vi "Server.vi"() -> ()   [LabVIEW 2020]
panel:
  out "Kitchen Door 2":bool
  out "Kitchen Door 1":bool
  out "Balcony Door 1":bool
  out "Bedroom 1 Door 1":bool
  out "Balcony Door 2":bool
  out "Bedroom 2 Door 1":bool
  out "Bedroom 1 Curtain 1":bool
  out "Bedroom 2 Curtain 1":bool
  out "Kitchen Light 1":bool
  out "Balcony Light 3":bool
  out "Balcony Light 2":bool
  out "Balcony Light 1":bool
  out "Bedroom 2 Light 1":bool
  out "Bedroom 1 Light 1":bool
  out "Master Bedroom Curtain 1":bool
  out "Master Bedroom AC 1":bool
  out "Master Bedroom Door 1":bool
  out "Master Bedroom Light 2":bool
  out "Master Bedroom Light 1":bool
  in  "Tab Control 2":enum32{"Page 1"}(tab)
  in  "WindowsMediaPlayer":refnum<k7>(container)
  out "Living Room Curtain 1":bool
  out "Living Room Door 1":bool
  in  "Tab Control":T1(tab)
  out "Light Rotation":bool
  out "Automatic Curtains":bool
  out "Time (Hour)":dbl
  out "Master Curtains":bool
  out "Master Doors":bool
  out "Master Lights":bool
  out "Adaptive Brightness":bool
  out "TV Brightness":dbl(slide) scale=0.0..6.0
  out "TV Fast Forward Reverse":bool
  out "TV Fast Forward":bool
  out "TV Channel 2":bool
  out "TV Channel 1":bool
  out "TV Pause":bool
  out "TV Play":bool
  out "TV On/Off":bool
  out "TV Volume":i32
  out "Balcony Alarm":bool
  out "Bedroom 2 Alarm":bool
  out "Bedroom 1 Alarm":bool
  out "Kitchen Alarm":bool
  out "Master Bedroom Alarm":bool
  out "Living Room Alarm":bool
  out "Living Room Temperature":dbl(slide) scale=10.0..40.0
  out "Room Brightness":dbl(slide) scale=0.0..6.0
  out "Living Room Light 1 Dim":bool
  out "Living Room Light 2 Dim":bool
  out "Master Bedroom Light 1 Dim":bool
  out "Master Bedroom Light 2 Dim":bool
  out "Master Bedroom Temperature":dbl(slide) scale=10.0..40.0
  out "Bedroom 1 Temperature":dbl(slide) scale=10.0..40.0
  out "Bedroom 1 Light 1 Dim":bool
  out "Bedroom 2 Temperature":dbl(slide) scale=10.0..40.0
  out "Bedroom 2 Light 1 Dim":bool
  out "Balcony Temperature":dbl(slide) scale=10.0..40.0
  out "Balcony Light 3 Dim":bool
  out "Balcony Light 2 Dim":bool
  out "Balcony Light 1 Dim":bool
  out "Kitchen Temperature":dbl(slide) scale=10.0..40.0
  out "Kitchen Light 1 Dim":bool
  out "Boolean":bool
  out "Living Room Light 2":bool
  out "Living Room Light 1":bool
  in  "stop":bool
  # "Server"
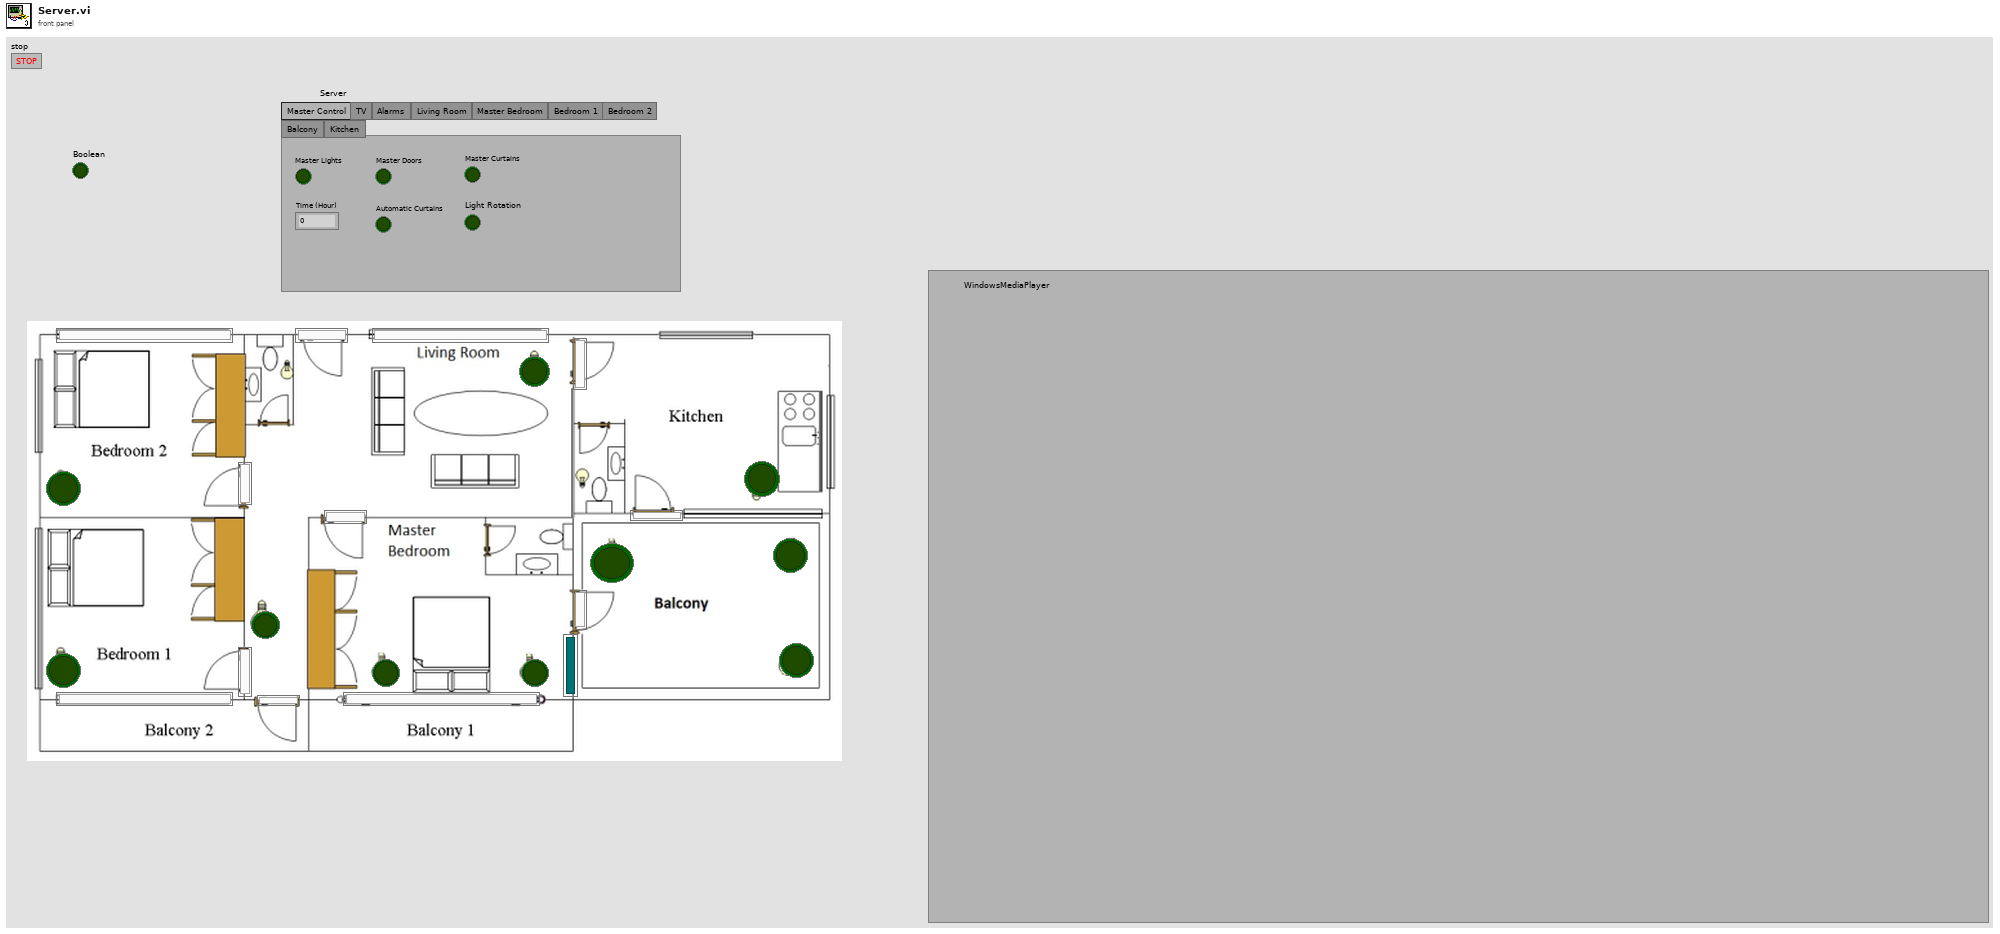
[diagram p1: front panel]
types:
  T1 = enum32{"Master Control", "TV", "Alarms", "Living Room", "Master Bedroom", "Bedroom 1", "Bedroom 2", "Balcony", "Kitchen"}
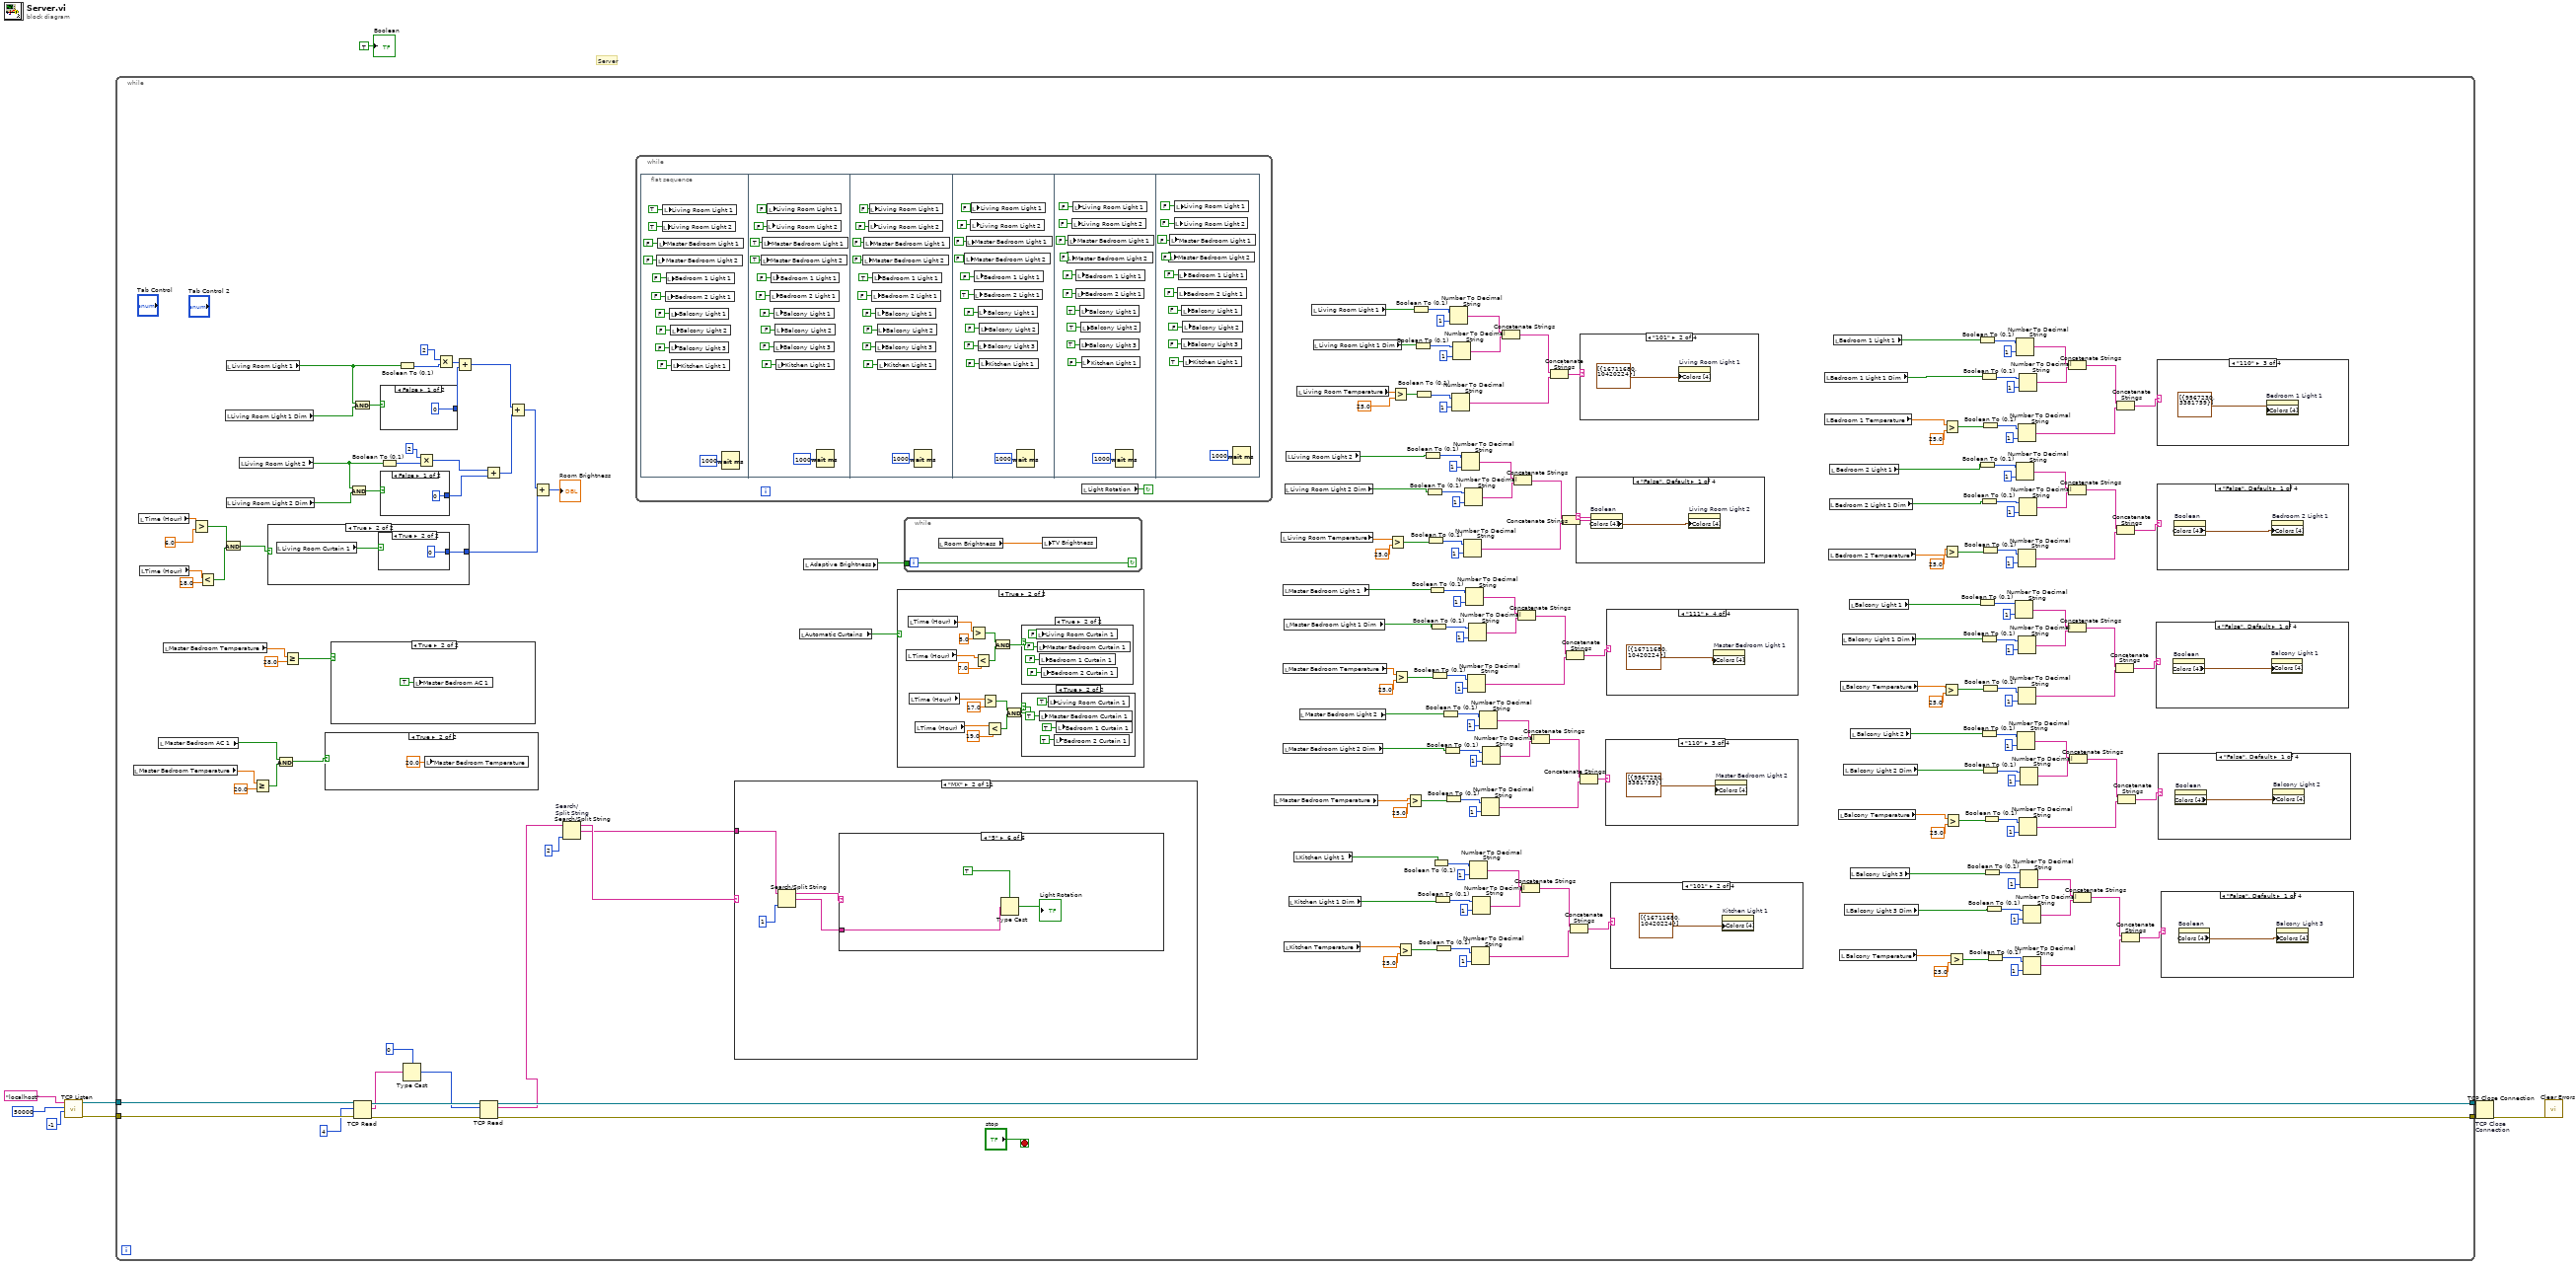
[diagram p0: block diagram]
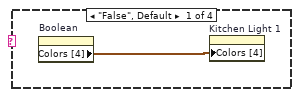
[diagram p2: hidden frame]
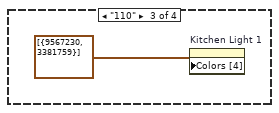
[diagram p3: hidden frame]
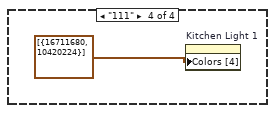
[diagram p4: hidden frame]
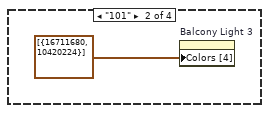
[diagram p5: hidden frame]
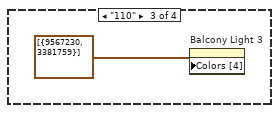
[diagram p6: hidden frame]
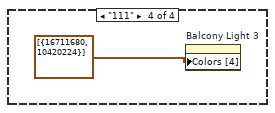
[diagram p7: hidden frame]
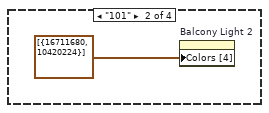
[diagram p8: hidden frame]
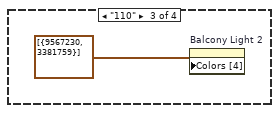
[diagram p9: hidden frame]
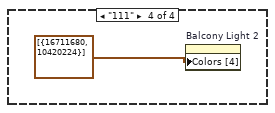
[diagram p10: hidden frame]
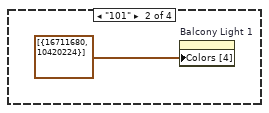
[diagram p11: hidden frame]
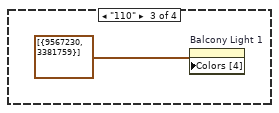
[diagram p12: hidden frame]
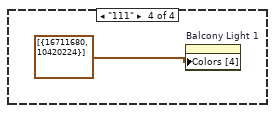
[diagram p13: hidden frame]
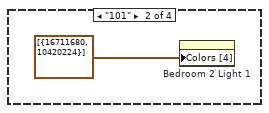
[diagram p14: hidden frame]
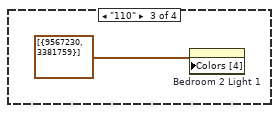
[diagram p15: hidden frame]
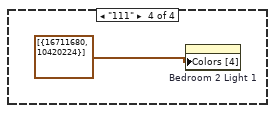
[diagram p16: hidden frame]
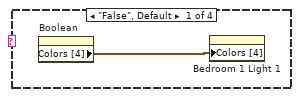
[diagram p17: hidden frame]
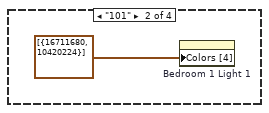
[diagram p18: hidden frame]
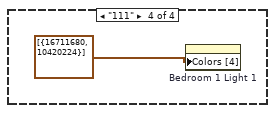
[diagram p19: hidden frame]
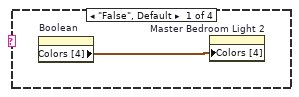
[diagram p20: hidden frame]
diagram:
  # "Server"
  n1 = call <vilib>:"TCP Listen.vi"("timeout ms (wait forever: -1)"=-1, "port"=u16 50000, "service name"="localhost") -> ("error out"=w4:errorcluster, "connection ID"=w6:refnum<k5>)  [unwired: 4 in, 3 out]
  n2 = while {
    tunnel: w6 -> [w219]
    tunnel: [w217] -> w5
    tunnel: w4 -> [w216]
    tunnel: [w214] -> w3
    stop <- "stop" stop-if-true
    n3 = local read "Master Bedroom Temperature"() -> (w141:dbl)
    n4 = local read "Time (Hour)"() -> (w154:dbl)
    n5 = local read "Time (Hour)"() -> (w152:dbl)
    n6 = local read "Master Bedroom AC 1"() -> (w142:bool)
    n7 = local read "Master Bedroom Temperature"() -> (w145:dbl)
    n8 = Greater?(x=w154, y=6.0) -> (0:w150:bool)
    n9 = Less?(x=w152, y=18.0) -> (x < y?=w149:bool)
    n10 = And(x=w150, y=w149) -> (x .and. y?=w148:bool)
    n11 = local read "Living Room Light 1 Dim"() -> (w192:bool)
    n12 = local read "Living Room Light 1"() -> (w193:bool)
    n13 = local read "Living Room Light 2 Dim"() -> (w189:bool)
    n14 = local read "Living Room Light 2"() -> (w188:bool)
    n15 = Greater Or Equal?(x=w141, y=20.0) -> (x >= y?=w139:bool)
    n16 = case shown="True" w148 {
      tunnel: [0 w347] -> w155
      frame False {
      }
      frame True {
        n17 = local read "Living Room Curtain 1"() -> (w348:bool)
        n18 = case shown="True" w348 {
          tunnel: [2 0] -> w347
          frame False {
          }
          frame True {
          }
        }
      }
    }
    n19 = And(x=w142, y=w139) -> (x .and. y?=w138:bool)
    n20 = Greater Or Equal?(x=w145, y=28.0) -> (x >= y?=w143:bool)
    n21 = case shown="True" w138 {
      frame False {
      }
      frame True {
        n22 = local write "Master Bedroom Temperature"(20.0 ("Master Bedroom Temperature")) -> ()
      }
    }
    n23 = case shown="True" w143 {
      frame False {
      }
      frame True {
        n24 = local write "Master Bedroom AC 1"(TRUE ("Master Bedroom AC 1")) -> ()
      }
    }
    n25 = And(x=w188, y=w189) -> (x .and. y?=w191:bool)
    n26 = And(x=w193, y=w192) -> (x .and. y?=w190:bool)
    n27 = TCP Read(connection ID=w219, bytes to read=4, error in (no error)=w216) -> (connection ID out=w218:refnum<k5>, data out=w212:string, error out=w215:errorcluster)  [unwired: 2 in]
    n28 = case shown="False" w190 {
      tunnel: [0 -1] -> w186
      frame False {
      }
      frame True {
      }
    }
    n29 = Boolean To (0,1)(Boolean=w188) -> (0, 1=w196:i16)
    n30 = case shown="False" w191 {
      tunnel: [0 -1] -> w187
      frame False {
      }
      frame True {
      }
    }
    n31 = Boolean To (0,1)(Boolean=w193) -> (0, 1=w198:i16)
    n32 = Type Cast(type=0 ("bytes to read"), x=w212) -> (*(type *) &x=w208:i32)
    n33 = Multiply(x=i16 2, y=w196) -> (x*y=w194:i16)
    n34 = Multiply(x=i16 2, y=w198) -> (x*y=w199:i16)
    n35 = Add(x=w199, y=w186) -> (x+y=w201:i32)
    n36 = TCP Read(connection ID=w218, bytes to read=w208, error in (no error)=w215) -> (connection ID out=w217:refnum<k5>, data out=w210:string, error out=w214:errorcluster)  [unwired: 2 in]
    n37 = Add(x=w194, y=w187) -> (x+y=w200:i32)
    n38 = Add(x=w201, y=w200) -> (x+y=w156:i32)
    n39 = Add(x=w156, y=w155) -> (x+y=→"Room Brightness":i32)
    n40 = Search/Split String "Search/\nSplit String"(string=w210, offset (0)=2) -> (substring before match=w207:string, match + rest of string=w206:string)  [unwired: 1 in, 1 out]
    n41 = while {
      stop <- w221 continue-if-true
      n42 = flat-sequence {
        frame #0 {
          n43 = local write "Master Bedroom Light 2"(FALSE ("Master Bedroom Light 2")) -> ()
          n44 = local write "Master Bedroom Light 1"(FALSE ("Master Bedroom Light 1")) -> ()
          n45 = local write "Living Room Light 2"(TRUE ("Living Room Light 2")) -> ()
          n46 = local write "Living Room Light 1"(TRUE ("Living Room Light 1")) -> ()
          n47 = local write "Bedroom 2 Light 1"(FALSE ("Bedroom 2 Light 1")) -> ()
          n48 = local write "Bedroom 1 Light 1"(FALSE ("Bedroom 1 Light 1")) -> ()
          n49 = local write "Balcony Light 1"(FALSE ("Balcony Light 1")) -> ()
          n50 = local write "Balcony Light 3"(FALSE ("Balcony Light 3")) -> ()
          n51 = local write "Balcony Light 2"(FALSE ("Balcony Light 2")) -> ()
          n52 = local write "Kitchen Light 1"(FALSE ("Kitchen Light 1")) -> ()
          n53 = Wait (ms)(milliseconds to wait=u32 1000) -> ()  [unwired: 1 out]
        }
        frame #1 {
          n54 = local write "Master Bedroom Light 2"(TRUE ("Master Bedroom Light 2")) -> ()
          n55 = local write "Master Bedroom Light 1"(TRUE ("Master Bedroom Light 1")) -> ()
          n56 = local write "Living Room Light 2"(FALSE ("Living Room Light 2")) -> ()
          n57 = local write "Living Room Light 1"(FALSE ("Living Room Light 1")) -> ()
          n58 = local write "Bedroom 2 Light 1"(FALSE ("Bedroom 2 Light 1")) -> ()
          n59 = local write "Bedroom 1 Light 1"(FALSE ("Bedroom 1 Light 1")) -> ()
          n60 = local write "Balcony Light 1"(FALSE ("Balcony Light 1")) -> ()
          n61 = local write "Balcony Light 3"(FALSE ("Balcony Light 3")) -> ()
          n62 = local write "Balcony Light 2"(FALSE ("Balcony Light 2")) -> ()
          n63 = local write "Kitchen Light 1"(FALSE ("Kitchen Light 1")) -> ()
          n64 = Wait (ms)(milliseconds to wait=u32 1000) -> ()  [unwired: 1 out]
        }
        frame #2 {
          n65 = local write "Master Bedroom Light 2"(FALSE ("Master Bedroom Light 2")) -> ()
          n66 = local write "Master Bedroom Light 1"(FALSE ("Master Bedroom Light 1")) -> ()
          n67 = local write "Living Room Light 2"(FALSE ("Living Room Light 2")) -> ()
          n68 = local write "Living Room Light 1"(FALSE ("Living Room Light 1")) -> ()
          n69 = local write "Bedroom 2 Light 1"(FALSE ("Bedroom 2 Light 1")) -> ()
          n70 = local write "Bedroom 1 Light 1"(TRUE ("Bedroom 1 Light 1")) -> ()
          n71 = local write "Balcony Light 1"(FALSE ("Balcony Light 1")) -> ()
          n72 = local write "Balcony Light 3"(FALSE ("Balcony Light 3")) -> ()
          n73 = local write "Balcony Light 2"(FALSE ("Balcony Light 2")) -> ()
          n74 = local write "Kitchen Light 1"(FALSE ("Kitchen Light 1")) -> ()
          n75 = Wait (ms)(milliseconds to wait=u32 1000) -> ()  [unwired: 1 out]
        }
        frame #3 {
          n76 = local write "Master Bedroom Light 2"(FALSE ("Master Bedroom Light 2")) -> ()
          n77 = local write "Master Bedroom Light 1"(FALSE ("Master Bedroom Light 1")) -> ()
          n78 = local write "Living Room Light 2"(FALSE ("Living Room Light 2")) -> ()
          n79 = local write "Living Room Light 1"(FALSE ("Living Room Light 1")) -> ()
          n80 = local write "Bedroom 2 Light 1"(TRUE ("Bedroom 2 Light 1")) -> ()
          n81 = local write "Bedroom 1 Light 1"(FALSE ("Bedroom 1 Light 1")) -> ()
          n82 = local write "Balcony Light 1"(FALSE ("Balcony Light 1")) -> ()
          n83 = local write "Balcony Light 3"(FALSE ("Balcony Light 3")) -> ()
          n84 = local write "Balcony Light 2"(FALSE ("Balcony Light 2")) -> ()
          n85 = local write "Kitchen Light 1"(FALSE ("Kitchen Light 1")) -> ()
          n86 = Wait (ms)(milliseconds to wait=u32 1000) -> ()  [unwired: 1 out]
        }
        frame #4 {
          n87 = local write "Master Bedroom Light 2"(FALSE ("Master Bedroom Light 2")) -> ()
          n88 = local write "Master Bedroom Light 1"(FALSE ("Master Bedroom Light 1")) -> ()
          n89 = local write "Living Room Light 2"(FALSE ("Living Room Light 2")) -> ()
          n90 = local write "Living Room Light 1"(FALSE ("Living Room Light 1")) -> ()
          n91 = local write "Bedroom 2 Light 1"(FALSE ("Bedroom 2 Light 1")) -> ()
          n92 = local write "Bedroom 1 Light 1"(FALSE ("Bedroom 1 Light 1")) -> ()
          n93 = local write "Balcony Light 1"(TRUE ("Balcony Light 1")) -> ()
          n94 = local write "Balcony Light 3"(TRUE ("Balcony Light 3")) -> ()
          n95 = local write "Balcony Light 2"(TRUE ("Balcony Light 2")) -> ()
          n96 = local write "Kitchen Light 1"(FALSE ("Kitchen Light 1")) -> ()
          n97 = Wait (ms)(milliseconds to wait=u32 1000) -> ()  [unwired: 1 out]
        }
        frame #5 {
          n98 = local write "Master Bedroom Light 2"(FALSE ("Master Bedroom Light 2")) -> ()
          n99 = local write "Master Bedroom Light 1"(FALSE ("Master Bedroom Light 1")) -> ()
          n100 = local write "Living Room Light 2"(FALSE ("Living Room Light 2")) -> ()
          n101 = local write "Living Room Light 1"(FALSE ("Living Room Light 1")) -> ()
          n102 = local write "Bedroom 2 Light 1"(FALSE ("Bedroom 2 Light 1")) -> ()
          n103 = local write "Bedroom 1 Light 1"(FALSE ("Bedroom 1 Light 1")) -> ()
          n104 = local write "Balcony Light 1"(FALSE ("Balcony Light 1")) -> ()
          n105 = local write "Balcony Light 3"(FALSE ("Balcony Light 3")) -> ()
          n106 = local write "Balcony Light 2"(FALSE ("Balcony Light 2")) -> ()
          n107 = local write "Kitchen Light 1"(TRUE ("Kitchen Light 1")) -> ()
          n108 = Wait (ms)(milliseconds to wait=u32 1000) -> ()  [unwired: 1 out]
        }
      }
      n109 = local read "Light Rotation"() -> (w221:bool)
    }
    n110 = case shown="\"MX\"" w207 {
      tunnel: w206 -> [_ w363 w387 w450 w487 w528 w556 w584 w632 w658 w685]
      frame "False", Default {
      }
      frame "MX" {
        n111 = Search/Split String(string=w363, offset (0)=1) -> (substring before match=w366:string, match + rest of string=w365:string)  [unwired: 1 in, 1 out]
        n112 = case shown="\"5\"" w366 {
          tunnel: w365 -> [_ w369 w371 w373 w377 w379]
          frame "False", Default {
          }
          frame "1" {
            n113 = Type Cast(type=TRUE, x=w369) -> (*(type *) &x=→"Master Lights":bool)
          }
          frame "2" {
            n114 = Type Cast(type=TRUE, x=w371) -> (*(type *) &x=→"Master Doors":bool)
          }
          frame "3" {
            n115 = Type Cast(type=TRUE, x=w373) -> (*(type *) &x=→"Master Curtains":bool)
          }
          frame "4" {
            n116 = Type Cast(type=TRUE, x=w377) -> (*(type *) &x=→"Automatic Curtains":bool)
          }
          frame "5" {
            n117 = Type Cast(type=TRUE, x=w379) -> (*(type *) &x=→"Light Rotation":bool)
          }
        }
      }
      frame "TV" {
        n118 = property on="WindowsMediaPlayer" class="AXCont"("Height"=u32 360 ("Container Bounds:Height")) -> ()  [unwired: 2 in, 2 out]
        n119 = property on="WindowsMediaPlayer" class="AXCont"("Width"=u32 640 ("Container Bounds:Width")) -> ()  [unwired: 2 in, 2 out]
        n120 = Search/Split String(string=w387, offset (0)=1) -> (substring before match=w386:string, match + rest of string=w385:string)  [unwired: 1 in, 1 out]
        n121 = case shown="\"1\"" w386 {
          tunnel: w385 -> [_ w390 w397 w403 w410 w418 w424 w431 w440 w442 w445]
          tunnel: "WindowsMediaPlayer" -> [_ _ w394 w402 w409 w413 w422 w430 w436 _ _]
          frame "False", Default {
          }
          frame "1" {
            n122 = Type Cast(type=TRUE, x=w390) -> (*(type *) &x=w389:bool)
            "TV On/Off" <- w389
            n123 = property on="WindowsMediaPlayer" class="AXCont"("Visible"=w389) -> ()  [unwired: 2 in, 2 out]
          }
          frame "2" {
            n124 = Automation Open(Automation Refnum=w394) -> (Automation Refnum=w395:refnum<k7>)  [unwired: 3 in, 1 out]
            n125 = property class="IWMPPlayer4"(reference=w395) -> ("controls"=w393:refnum<k7>)  [unwired: 1 in, 2 out]
            n126 = Type Cast(type=TRUE, x=w397) -> (*(type *) &x=→"TV Play":bool)
            n127 = invoke class="IWMPControls" method="play"(reference=w393) -> (reference out=w392:refnum<k7>)  [unwired: 2 in, 2 out]
            n128 = Close Reference(reference=w392) -> ()  [unwired: 1 in, 1 out]
          }
          frame "3" {
            n129 = Automation Open(Automation Refnum=w402) -> (Automation Refnum=w401:refnum<k7>)  [unwired: 3 in, 1 out]
            n130 = property class="IWMPPlayer4"(reference=w401) -> ("controls"=w400:refnum<k7>)  [unwired: 1 in, 2 out]
            n131 = Type Cast(type=TRUE, x=w403) -> (*(type *) &x=→"TV Pause":bool)
            n132 = invoke class="IWMPControls" method="pause"(reference=w400) -> (reference out=w399:refnum<k7>)  [unwired: 2 in, 2 out]
            n133 = Close Reference(reference=w399) -> ()  [unwired: 1 in, 1 out]
          }
          frame "4" {
            n134 = Automation Open(Automation Refnum=w409) -> (Automation Refnum=w408:refnum<k7>)  [unwired: 3 in, 1 out]
            n135 = property class="IWMPPlayer4"(reference=w408, "URL"="C:/Ah ! Guilty Gear !!.mp4") -> (reference out=w407:refnum<k7>)  [unwired: 1 in, 1 out]
            n136 = Type Cast(type=TRUE, x=w410) -> (*(type *) &x=→"TV Channel 1":bool)
            n137 = Close Reference(reference=w407) -> ()  [unwired: 1 in, 1 out]
          }
          frame "5" {
            n138 = Automation Open(Automation Refnum=w413) -> (Automation Refnum=w414:refnum<k7>)  [unwired: 3 in, 1 out]
            n139 = property class="IWMPPlayer4"(reference=w414, "URL"="C:/TIME2REALIZE.mp4") -> (reference out=w415:refnum<k7>)  [unwired: 1 in, 1 out]
            n140 = Type Cast(type=TRUE, x=w418) -> (*(type *) &x=→"TV Channel 2":bool)
            n141 = Close Reference(reference=w415) -> ()  [unwired: 1 in, 1 out]
          }
          frame "6" {
            n142 = Automation Open(Automation Refnum=w422) -> (Automation Refnum=w421:refnum<k7>)  [unwired: 3 in, 1 out]
            n143 = property class="IWMPPlayer4"(reference=w421) -> ("controls"=w423:refnum<k7>)  [unwired: 1 in, 2 out]
            n144 = Type Cast(type=TRUE, x=w424) -> (*(type *) &x=→"TV Fast Forward":bool)
            n145 = invoke class="IWMPControls" method="fastForward"(reference=w423) -> (reference out=w420:refnum<k7>)  [unwired: 2 in, 2 out]
            n146 = Close Reference(reference=w420) -> ()  [unwired: 1 in, 1 out]
          }
          frame "7" {
            n147 = Automation Open(Automation Refnum=w430) -> (Automation Refnum=w429:refnum<k7>)  [unwired: 3 in, 1 out]
            n148 = property class="IWMPPlayer4"(reference=w429) -> ("controls"=w428:refnum<k7>)  [unwired: 1 in, 2 out]
            n149 = Type Cast(type=TRUE, x=w431) -> (*(type *) &x=→"TV Fast Forward Reverse":bool)
            n150 = invoke class="IWMPControls" method="fastReverse"(reference=w428) -> (reference out=w427:refnum<k7>)  [unwired: 2 in, 2 out]
            n151 = Close Reference(reference=w427) -> ()  [unwired: 1 in, 1 out]
          }
          frame "8" {
            n152 = Automation Open(Automation Refnum=w436) -> (Automation Refnum=w435:refnum<k7>)  [unwired: 3 in, 1 out]
            n153 = property class="IWMPPlayer4"(reference=w435) -> ("settings"=w437:refnum<k7>)  [unwired: 1 in, 2 out]
            n154 = Type Cast(type=0, x=w440) -> (*(type *) &x=w438:i32)
            "TV Volume" <- w438
            n155 = property class="IWMPSettings"(reference=w437, "volume"=w438) -> (reference out=w434:refnum<k7>)  [unwired: 1 in, 1 out]
            n156 = Close Reference(reference=w434) -> ()  [unwired: 1 in, 1 out]
          }
          frame "9" {
            n157 = Type Cast(type=0.0, x=w442) -> (*(type *) &x=→"TV Brightness":dbl)
          }
          frame "10" {
            n158 = Type Cast(type=TRUE, x=w445) -> (*(type *) &x=→"Adaptive Brightness":bool)
          }
        }
      }
      frame "LR" {
        n159 = Search/Split String(string=w450, offset (0)=1) -> (substring before match=w448:string, match + rest of string=w447:string)  [unwired: 1 in, 1 out]
        n160 = case shown="\"1\"" w448 {
          tunnel: w447 -> [_ w453 w460 w466 w469 w473 w480]
          frame "False", Default {
          }
          frame "1" {
            n161 = local read "Master Lights"() -> (w452:bool)
            n162 = Not(x=w452) -> (.not. x?=w451:bool)
            n163 = case shown="True" w451 {
              tunnel: w453 -> [_ w455]
              frame False {
                n164 = local write "Living Room Alarm"(TRUE ("Living Room Alarm")) -> ()
              }
              frame True {
                n165 = Type Cast(type=FALSE ("Boolean"), x=w455) -> (*(type *) &x=→"Living Room Light 1":bool)
              }
            }
          }
          frame "2" {
            n166 = local read "Master Lights"() -> (w459:bool)
            n167 = Not(x=w459) -> (.not. x?=w458:bool)
            n168 = case shown="True" w458 {
              tunnel: w460 -> [_ w462]
              frame False {
                n169 = local write "Living Room Alarm"(TRUE ("Living Room Alarm")) -> ()
              }
              frame True {
                n170 = Type Cast(type=FALSE ("Boolean"), x=w462) -> (*(type *) &x=→"Living Room Light 2":bool)
              }
            }
          }
          frame "3" {
            n171 = Type Cast(type=FALSE ("Boolean"), x=w466) -> (*(type *) &x=→"Living Room Light 1 Dim":bool)
          }
          frame "4" {
            n172 = Type Cast(type=FALSE ("Boolean"), x=w469) -> (*(type *) &x=→"Living Room Light 2 Dim":bool)
          }
          frame "5" {
            n173 = local read "Master Curtains"() -> (w472:bool)
            n174 = Not(x=w472) -> (.not. x?=w471:bool)
            n175 = case shown="True" w471 {
              tunnel: w473 -> [_ w477]
              frame False {
                n176 = local write "Living Room Alarm"(TRUE ("Living Room Alarm")) -> ()
              }
              frame True {
                n177 = Type Cast(type=TRUE, x=w477) -> (*(type *) &x=→"Living Room Curtain 1":bool)
              }
            }
          }
          frame "6" {
            n178 = local read "Master Doors"() -> (w479:bool)
            n179 = Not(x=w479) -> (.not. x?=w478:bool)
            n180 = case shown="False" w478 {
              tunnel: w480 -> [_ w482]
              frame False {
                n181 = local write "Living Room Alarm"(TRUE ("Living Room Alarm")) -> ()
              }
              frame True {
                n182 = Type Cast(type=FALSE ("Boolean"), x=w482) -> (*(type *) &x=→"Living Room Door 1":bool)
              }
            }
          }
        }
      }
      frame "MB" {
        n183 = Search/Split String(string=w487, offset (0)=1) -> (substring before match=w486:string, match + rest of string=w485:string)  [unwired: 1 in, 1 out]
        n184 = case shown="\"5\"" w486 {
          tunnel: w485 -> [_ w489 w498 w504 w507 w511 w516 w524]
          frame "False", Default {
          }
          frame "1" {
            n185 = local read "Master Lights"() -> (w491:bool)
            n186 = Not(x=w491) -> (.not. x?=w490:bool)
            n187 = case shown="True" w490 {
              tunnel: w489 -> [_ w494]
              frame False {
                n188 = local write "Master Bedroom Alarm"(TRUE ("Master Bedroom Alarm")) -> ()
              }
              frame True {
                n189 = Type Cast(type=FALSE ("Boolean"), x=w494) -> (*(type *) &x=→"Master Bedroom Light 1":bool)
              }
            }
          }
          frame "2" {
            n190 = local read "Master Lights"() -> (w497:bool)
            n191 = Not(x=w497) -> (.not. x?=w496:bool)
            n192 = case shown="False" w496 {
              tunnel: w498 -> [_ w501]
              frame False {
                n193 = local write "Master Bedroom Alarm"(TRUE ("Master Bedroom Alarm")) -> ()
              }
              frame True {
                n194 = Type Cast(type=FALSE ("Boolean"), x=w501) -> (*(type *) &x=→"Master Bedroom Light 2":bool)
              }
            }
          }
          frame "3" {
            n195 = Type Cast(type=FALSE ("Boolean"), x=w504) -> (*(type *) &x=→"Master Bedroom Light 1 Dim":bool)
          }
          frame "4" {
            n196 = Type Cast(type=FALSE ("Boolean"), x=w507) -> (*(type *) &x=→"Master Bedroom Light 2 Dim":bool)
          }
          frame "5" {
            n197 = local read "Master Curtains"() -> (w510:bool)
            n198 = Not(x=w510) -> (.not. x?=w509:bool)
            n199 = case shown="True" w509 {
              tunnel: w511 -> [_ w514]
              frame False {
                n200 = local write "Master Bedroom Alarm"(TRUE ("Master Bedroom Alarm")) -> ()
              }
              frame True {
                n201 = Type Cast(type=FALSE ("Boolean"), x=w514) -> (*(type *) &x=→"Master Bedroom Curtain 1":bool)
              }
            }
          }
          frame "6" {
            n202 = local read "Master Doors"() -> (w518:bool)
            n203 = Not(x=w518) -> (.not. x?=w517:bool)
            n204 = case shown="True" w517 {
              tunnel: w516 -> [_ w521]
              frame False {
                n205 = local write "Master Bedroom Alarm"(TRUE ("Master Bedroom Alarm")) -> ()
              }
              frame True {
                n206 = Type Cast(type=FALSE ("Boolean"), x=w521) -> (*(type *) &x=→"Master Bedroom Door 1":bool)
              }
            }
          }
          frame "7" {
            n207 = Type Cast(type=FALSE ("Boolean"), x=w524) -> (*(type *) &x=→"Master Bedroom AC 1":bool)
          }
        }
      }
      frame "B1" {
        n208 = Search/Split String(string=w528, offset (0)=1) -> (substring before match=w527:string, match + rest of string=w526:string)  [unwired: 1 in, 1 out]
        n209 = case shown="\"3\"" w527 {
          tunnel: w526 -> [_ w532 w538 w540 w547]
          frame "False", Default {
          }
          frame "1" {
            n210 = local read "Master Lights"() -> (w531:bool)
            n211 = Not(x=w531) -> (.not. x?=w530:bool)
            n212 = case shown="True" w530 {
              tunnel: w532 -> [_ w534]
              frame False {
                n213 = local write "Bedroom 1 Alarm"(TRUE ("Bedroom 1 Alarm")) -> ()
              }
              frame True {
                n214 = Type Cast(type=TRUE, x=w534) -> (*(type *) &x=→"Bedroom 1 Light 1":bool)
              }
            }
          }
          frame "2" {
            n215 = Type Cast(type=TRUE, x=w538) -> (*(type *) &x=→"Bedroom 1 Light 1 Dim":bool)
          }
          frame "3" {
            n216 = local read "Master Curtains"() -> (w542:bool)
            n217 = Not(x=w542) -> (.not. x?=w541:bool)
            n218 = case shown="True" w541 {
              tunnel: w540 -> [_ w544]
              frame False {
                n219 = local write "Bedroom 1 Alarm"(TRUE ("Bedroom 1 Alarm")) -> ()
              }
              frame True {
                n220 = Type Cast(type=FALSE ("Boolean"), x=w544) -> (*(type *) &x=→"Bedroom 1 Curtain 1":bool)
              }
            }
          }
          frame "4" {
            n221 = local read "Master Doors"() -> (w548:bool)
            n222 = Not(x=w548) -> (.not. x?=w549:bool)
            n223 = case shown="False" w549 {
              tunnel: w547 -> [_ w551]
              frame False {
                n224 = local write "Bedroom 1 Alarm"(TRUE ("Bedroom 1 Alarm")) -> ()
              }
              frame True {
                n225 = Type Cast(type=FALSE ("Boolean"), x=w551) -> (*(type *) &x=→"Bedroom 1 Door 1":bool)
              }
            }
          }
        }
      }
      frame "B2" {
        n226 = Search/Split String(string=w556, offset (0)=1) -> (substring before match=w555:string, match + rest of string=w554:string)  [unwired: 1 in, 1 out]
        n227 = case shown="\"4\"" w555 {
          tunnel: w554 -> [_ w560 w565 w568 w577]
          frame "False", Default {
          }
          frame "1" {
            n228 = local read "Master Lights"() -> (w558:bool)
            n229 = Not(x=w558) -> (.not. x?=w559:bool)
            n230 = case shown="True" w559 {
              tunnel: w560 -> [_ w563]
              frame False {
                n231 = local write "Bedroom 2 Alarm"(TRUE ("Bedroom 2 Alarm")) -> ()
              }
              frame True {
                n232 = Type Cast(type=TRUE, x=w563) -> (*(type *) &x=→"Bedroom 2 Light 1":bool)
              }
            }
          }
          frame "2" {
            n233 = Type Cast(type=TRUE, x=w565) -> (*(type *) &x=→"Bedroom 2 Light 1 Dim":bool)
          }
          frame "3" {
            n234 = local read "Master Curtains"() -> (w570:bool)
            n235 = Not(x=w570) -> (.not. x?=w569:bool)
            n236 = case shown="False" w569 {
              tunnel: w568 -> [_ w572]
              frame False {
                n237 = local write "Bedroom 2 Alarm"(TRUE ("Bedroom 2 Alarm")) -> ()
              }
              frame True {
                n238 = Type Cast(type=FALSE ("Boolean"), x=w572) -> (*(type *) &x=→"Bedroom 2 Curtain 1":bool)
              }
            }
          }
          frame "4" {
            n239 = local read "Master Doors"() -> (w576:bool)
            n240 = Not(x=w576) -> (.not. x?=w575:bool)
            n241 = case shown="False" w575 {
              tunnel: w577 -> [_ w579]
              frame False {
                n242 = local write "Bedroom 2 Alarm"(TRUE ("Bedroom 2 Alarm")) -> ()
              }
              frame True {
                n243 = Type Cast(type=FALSE ("Boolean"), x=w579) -> (*(type *) &x=→"Bedroom 2 Door 1":bool)
              }
            }
          }
        }
      }
      frame "BA" {
        n244 = Search/Split String(string=w584, offset (0)=1) -> (substring before match=w583:string, match + rest of string=w582:string)  [unwired: 1 in, 1 out]
        n245 = case shown="\"1\"" w583 {
          tunnel: w582 -> [_ w588 w595 w602 w607 w610 w613 w618 w625]
          frame "False", Default {
          }
          frame "1" {
            n246 = local read "Master Lights"() -> (w586:bool)
            n247 = Not(x=w586) -> (.not. x?=w587:bool)
            n248 = case shown="True" w587 {
              tunnel: w588 -> [_ w590]
              frame False {
                n249 = local write "Balcony Alarm"(TRUE ("Balcony Alarm")) -> ()
              }
              frame True {
                n250 = Type Cast(type=TRUE, x=w590) -> (*(type *) &x=→"Balcony Light 1":bool)
              }
            }
          }
          frame "2" {
            n251 = local read "Master Lights"() -> (w594:bool)
            n252 = Not(x=w594) -> (.not. x?=w593:bool)
            n253 = case shown="False" w593 {
              tunnel: w595 -> [_ w597]
              frame False {
                n254 = local write "Balcony Alarm"(TRUE ("Balcony Alarm")) -> ()
              }
              frame True {
                n255 = Type Cast(type=TRUE, x=w597) -> (*(type *) &x=→"Balcony Light 2":bool)
              }
            }
          }
          frame "3" {
            n256 = local read "Master Lights"() -> (w600:bool)
            n257 = Not(x=w600) -> (.not. x?=w601:bool)
            n258 = case shown="False" w601 {
              tunnel: w602 -> [_ w604]
              frame False {
                n259 = local write "Balcony Alarm"(TRUE ("Balcony Alarm")) -> ()
              }
              frame True {
                n260 = Type Cast(type=TRUE, x=w604) -> (*(type *) &x=→"Balcony Light 3":bool)
              }
            }
          }
          frame "4" {
            n261 = Type Cast(type=FALSE ("Boolean"), x=w607) -> (*(type *) &x=→"Balcony Light 1 Dim":bool)
          }
          frame "5" {
            n262 = Type Cast(type=FALSE ("Boolean"), x=w610) -> (*(type *) &x=→"Balcony Light 2 Dim":bool)
          }
          frame "6" {
            n263 = Type Cast(type=FALSE ("Boolean"), x=w613) -> (*(type *) &x=→"Balcony Light 3 Dim":bool)
          }
          frame "7" {
            n264 = local read "Master Doors"() -> (w617:bool)
            n265 = Not(x=w617) -> (.not. x?=w616:bool)
            n266 = case shown="False" w616 {
              tunnel: w618 -> [_ w620]
              frame False {
                n267 = local write "Balcony Alarm"(TRUE) -> ()
              }
              frame True {
                n268 = Type Cast(type=FALSE ("Boolean"), x=w620) -> (*(type *) &x=→"Balcony Door 1":bool)
              }
            }
          }
          frame "8" {
            n269 = local read "Balcony Alarm"() -> (w624:bool)
            n270 = Not(x=w624) -> (.not. x?=w623:bool)
            n271 = case shown="False" w623 {
              tunnel: w625 -> [_ w627]
              frame False {
                n272 = local write "Balcony Alarm"(TRUE ("Balcony Alarm")) -> ()
              }
              frame True {
                n273 = Type Cast(type=FALSE ("Boolean"), x=w627) -> (*(type *) &x=→"Balcony Door 2":bool)
              }
            }
          }
        }
      }
      frame "KI" {
        n274 = Search/Split String(string=w632, offset (0)=1) -> (substring before match=w631:string, match + rest of string=w630:string)  [unwired: 1 in, 1 out]
        n275 = case shown="\"1\"" w631 {
          tunnel: w630 -> [_ w636 w642 w646 w653]
          frame "False", Default {
          }
          frame "1" {
            n276 = local read "Master Lights"() -> (w635:bool)
            n277 = Not(x=w635) -> (.not. x?=w634:bool)
            n278 = case shown="True" w634 {
              tunnel: w636 -> [_ w638]
              frame False {
                n279 = local write "Kitchen Alarm"(TRUE ("Kitchen Alarm")) -> ()
              }
              frame True {
                n280 = Type Cast(type=TRUE, x=w638) -> (*(type *) &x=→"Kitchen Light 1":bool)
              }
            }
          }
          frame "2" {
            n281 = Type Cast(type=FALSE ("Boolean"), x=w642) -> (*(type *) &x=→"Kitchen Light 1 Dim":bool)
          }
          frame "3" {
            n282 = local read "Master Doors"() -> (w645:bool)
            n283 = Not(x=w645) -> (.not. x?=w644:bool)
            n284 = case shown="False" w644 {
              tunnel: w646 -> [_ w648]
              frame False {
                n285 = local write "Kitchen Alarm"(TRUE ("Kitchen Alarm")) -> ()
              }
              frame True {
                n286 = Type Cast(type=FALSE ("Boolean"), x=w648) -> (*(type *) &x=→"Kitchen Door 1":bool)
              }
            }
          }
          frame "4" {
            n287 = local read "Master Doors"() -> (w652:bool)
            n288 = Not(x=w652) -> (.not. x?=w651:bool)
            n289 = case shown="False" w651 {
              tunnel: w653 -> [_ w655]
              frame False {
                n290 = local write "Kitchen Alarm"(TRUE ("Kitchen Alarm")) -> ()
              }
              frame True {
                n291 = Type Cast(type=FALSE ("Boolean"), x=w655) -> (*(type *) &x=→"Kitchen Door 2":bool)
              }
            }
          }
        }
      }
      frame "HX" {
        n292 = Search/Split String(string=w658, offset (0)=1) -> (substring before match=w660:string, match + rest of string=w661:string)  [unwired: 1 in, 1 out]
        n293 = case shown="\"4\"" w660 {
          tunnel: w661 -> [_ w662 w666 w669 w671 w674 w677 w680]
          frame "False", Default {
          }
          frame "1" {
            n294 = Type Cast(type=0.0, x=w662) -> (*(type *) &x=→"Living Room Temperature":dbl)
          }
          frame "2" {
            n295 = Type Cast(type=0.0, x=w666) -> (*(type *) &x=→"Time (Hour)":dbl)
          }
          frame "3" {
            n296 = Type Cast(type=0.0, x=w669) -> (*(type *) &x=→"Master Bedroom Temperature":dbl)
          }
          frame "4" {
            n297 = Type Cast(type=0.0, x=w671) -> (*(type *) &x=→"Bedroom 1 Temperature":dbl)
          }
          frame "5" {
            n298 = Type Cast(type=0.0, x=w674) -> (*(type *) &x=→"Bedroom 2 Temperature":dbl)
          }
          frame "6" {
            n299 = Type Cast(type=0.0, x=w677) -> (*(type *) &x=→"Balcony Temperature":dbl)
          }
          frame "7" {
            n300 = Type Cast(type=0.0, x=w680) -> (*(type *) &x=→"Kitchen Temperature":dbl)
          }
        }
      }
      frame "AL" {
        n301 = Search/Split String(string=w685, offset (0)=1) -> (substring before match=w684:string, match + rest of string=w683:string)  [unwired: 1 in, 1 out]
        n302 = case shown="\"6\"" w684 {
          tunnel: w683 -> [_ w688 w691 w694 w696 w700 w702]
          frame "False", Default {
          }
          frame "1" {
            n303 = Type Cast(type=TRUE, x=w688) -> (*(type *) &x=→"Living Room Alarm":bool)
          }
          frame "2" {
            n304 = Type Cast(type=FALSE ("Boolean"), x=w691) -> (*(type *) &x=→"Master Bedroom Alarm":bool)
          }
          frame "3" {
            n305 = Type Cast(type=FALSE ("Boolean"), x=w694) -> (*(type *) &x=→"Bedroom 1 Alarm":bool)
          }
          frame "4" {
            n306 = Type Cast(type=FALSE ("Boolean"), x=w696) -> (*(type *) &x=→"Bedroom 2 Alarm":bool)
          }
          frame "5" {
            n307 = Type Cast(type=FALSE ("Boolean"), x=w700) -> (*(type *) &x=→"Balcony Alarm":bool)
          }
          frame "6" {
            n308 = Type Cast(type=FALSE ("Boolean"), x=w702) -> (*(type *) &x=→"Kitchen Alarm":bool)
          }
        }
      }
    }
    n309 = local read "Automatic Curtains"() -> (w147:bool)
    n310 = local read "Adaptive Brightness"() -> (w146:bool)
    n311 = case shown="True" w147 {
      frame False {
      }
      frame True {
        n312 = local read "Time (Hour)"() -> (w335:dbl)
        n313 = local read "Time (Hour)"() -> (w337:dbl)
        n314 = local read "Time (Hour)"() -> (w324:dbl)
        n315 = local read "Time (Hour)"() -> (w325:dbl)
        n316 = Greater?(x=w337, y=5.0) -> (0:w333:bool)
        n317 = Less?(x=w335, y=7.0) -> (x < y?=w332:bool)
        n318 = Greater?(x=w324, y=17.0) -> (0:w328:bool)
        n319 = Less?(x=w325, y=19.0) -> (x < y?=w327:bool)
        n320 = And(x=w333, y=w332) -> (x .and. y?=w331:bool)
        n321 = And(x=w328, y=w327) -> (x .and. y?=w326:bool)
        n322 = case shown="True" w331 {
          frame False {
          }
          frame True {
            n323 = local write "Living Room Curtain 1"(FALSE ("Living Room Curtain")) -> ()
            n324 = local write "Master Bedroom Curtain 1"(FALSE ("Master Bedroom Curtain 1")) -> ()
            n325 = local write "Bedroom 1 Curtain 1"(FALSE ("Bedroom 1 Curtain 1")) -> ()
            n326 = local write "Bedroom 2 Curtain 1"(FALSE ("Bedroom 2 Curtain 1")) -> ()
          }
        }
        n327 = case shown="True" w326 {
          frame False {
          }
          frame True {
            n328 = local write "Master Bedroom Curtain 1"(TRUE ("Master Bedroom Curtain 1")) -> ()
            n329 = local write "Living Room Curtain 1"(TRUE ("Living Room Curtain")) -> ()
            n330 = local write "Bedroom 2 Curtain 1"(TRUE ("Bedroom 2 Curtain 1")) -> ()
            n331 = local write "Bedroom 1 Curtain 1"(TRUE ("Bedroom 1 Curtain 1")) -> ()
          }
        }
      }
    }
    n332 = while {
      tunnel: w146 -> [w323]
      stop <- w323 continue-if-true
      n333 = local read "Room Brightness"() -> (w322:dbl)
      n334 = local write "TV Brightness"(w322) -> ()
    }
    n335 = local read "Master Bedroom Temperature"() -> (w93:dbl)
    n336 = local read "Living Room Temperature"() -> (w204:dbl)
    n337 = local read "Master Bedroom Light 1"() -> (w96:bool)
    n338 = local read "Master Bedroom Temperature"() -> (w98:dbl)
    n339 = local read "Master Bedroom Light 2 Dim"() -> (w94:bool)
    n340 = local read "Master Bedroom Light 1 Dim"() -> (w97:bool)
    n341 = local read "Kitchen Temperature"() -> (w24:dbl)
    n342 = local read "Living Room Light 2 Dim"() -> (w160:bool)
    n343 = local read "Living Room Light 2"() -> (w161:bool)
    n344 = local read "Kitchen Light 1 Dim"() -> (w23:bool)
    n345 = local read "Kitchen Light 1"() -> (w22:bool)
    n346 = local read "Living Room Temperature"() -> (w202:dbl)
    n347 = local read "Master Bedroom Light 2"() -> (w95:bool)
    n348 = local read "Living Room Light 1"() -> (w183:bool)
    n349 = local read "Living Room Light 1 Dim"() -> (w185:bool)
    n350 = Greater?(x=w204, y=25.0) -> (0:w159:bool)
    n351 = Greater?(x=w202, y=25.0) -> (0:w184:bool)
    n352 = Greater?(x=w98, y=25.0) -> (0:w126:bool)
    n353 = Greater?(x=w24, y=25.0) -> (0:w26:bool)
    n354 = Greater?(x=w93, y=25.0) -> (0:w114:bool)
    n355 = Boolean To (0,1)(Boolean=w183) -> (0, 1=w178:i16)
    n356 = Boolean To (0,1)(Boolean=w185) -> (0, 1=w181:i16)
    n357 = Boolean To (0,1)(Boolean=w184) -> (0, 1=w177:i16)
    n358 = Boolean To (0,1)(Boolean=w161) -> (0, 1=w167:i16)
    n359 = Boolean To (0,1)(Boolean=w160) -> (0, 1=w170:i16)
    n360 = Boolean To (0,1)(Boolean=w159) -> (0, 1=w166:i16)
    n361 = Boolean To (0,1)(Boolean=w96) -> (0, 1=w132:i16)
    n362 = Boolean To (0,1)(Boolean=w97) -> (0, 1=w135:i16)
    n363 = Boolean To (0,1)(Boolean=w126) -> (0, 1=w131:i16)
    n364 = Boolean To (0,1)(Boolean=w22) -> (0, 1=w32:i16)
    n365 = Boolean To (0,1)(Boolean=w23) -> (0, 1=w35:i16)
    n366 = Boolean To (0,1)(Boolean=w26) -> (0, 1=w31:i16)
    n367 = Boolean To (0,1)(Boolean=w95) -> (0, 1=w120:i16)
    n368 = Boolean To (0,1)(Boolean=w94) -> (0, 1=w123:i16)
    n369 = Boolean To (0,1)(Boolean=w114) -> (0, 1=w119:i16)
    n370 = Number To Decimal String(number=w178, width (-)=i16 1) -> (decimal integer string=w175:string)
    n371 = Number To Decimal String(number=w177, width (-)=i16 1) -> (decimal integer string=w173:string)
    n372 = Number To Decimal String(number=w181, width (-)=i16 1) -> (decimal integer string=w176:string)
    n373 = Number To Decimal String(number=w167, width (-)=i16 1) -> (decimal integer string=w164:string)
    n374 = Number To Decimal String(number=w166, width (-)=i16 1) -> (decimal integer string=w162:string)
    n375 = Number To Decimal String(number=w170, width (-)=i16 1) -> (decimal integer string=w165:string)
    n376 = Number To Decimal String(number=w132, width (-)=i16 1) -> (decimal integer string=w129:string)
    n377 = Number To Decimal String(number=w131, width (-)=i16 1) -> (decimal integer string=w127:string)
    n378 = Number To Decimal String(number=w135, width (-)=i16 1) -> (decimal integer string=w130:string)
    n379 = Number To Decimal String(number=w32, width (-)=i16 1) -> (decimal integer string=w29:string)
    n380 = Number To Decimal String(number=w31, width (-)=i16 1) -> (decimal integer string=w27:string)
    n381 = Number To Decimal String(number=w35, width (-)=i16 1) -> (decimal integer string=w30:string)
    n382 = Number To Decimal String(number=w120, width (-)=i16 1) -> (decimal integer string=w117:string)
    n383 = Number To Decimal String(number=w119, width (-)=i16 1) -> (decimal integer string=w115:string)
    n384 = Number To Decimal String(number=w123, width (-)=i16 1) -> (decimal integer string=w118:string)
    n385 = Concatenate Strings(w175, w176) -> (w174:string)
    n386 = Concatenate Strings(w164, w165) -> (w163:string)
    n387 = Concatenate Strings(w129, w130) -> (w128:string)
    n388 = Concatenate Strings(w29, w30) -> (w28:string)
    n389 = Concatenate Strings(w117, w118) -> (w116:string)
    n390 = Concatenate Strings(w174, w173) -> (w172:string)
    n391 = Concatenate Strings(w163, w162) -> (w158:string)
    n392 = Concatenate Strings(w128, w127) -> (w112:string)
    n393 = Concatenate Strings(w28, w27) -> (w25:string)
    n394 = case shown="\"False\", Default" w158 {
      frame "False", Default {
        n395 = property on="Boolean" class="Bool (strict)"() -> ("Colors [4]"=w351:cluster{u32, u32}[])  [unwired: 2 in, 2 out]
        n396 = property on="Living Room Light 2" class="Bool (strict)"("Colors [4]"=w351) -> ()  [unwired: 2 in, 2 out]
      }
      frame "101" {
        n397 = property on="Living Room Light 2" class="Bool (strict)"("Colors [4]"=cluster{u32, u32}[] [{16711680, 10420224}]) -> ()  [unwired: 2 in, 2 out]
      }
      frame "110" {
        n398 = property on="Living Room Light 2" class="Bool (strict)"("Colors [4]"=cluster{u32, u32}[] [{9567230, 3381759}]) -> ()  [unwired: 2 in, 2 out]
      }
      frame "111" {
        n399 = property on="Living Room Light 2" class="Bool (strict)"("Colors [4]"=cluster{u32, u32}[] [{16711680, 10420224}]) -> ()  [unwired: 2 in, 2 out]
      }
    }
    n400 = case shown="\"101\"" w172 {
      frame "False", Default {
        n401 = property on="Boolean" class="Bool (strict)"() -> ("Colors [4]"=w355:cluster{u32, u32}[])  [unwired: 2 in, 2 out]
        n402 = property on="Living Room Light 1" class="Bool (strict)"("Colors [4]"=w355) -> ()  [unwired: 2 in, 2 out]
      }
      frame "101" {
        n403 = property on="Living Room Light 1" class="Bool (strict)"("Colors [4]"=cluster{u32, u32}[] [{16711680, 10420224}]) -> ()  [unwired: 2 in, 2 out]
      }
      frame "110" {
        n404 = property on="Living Room Light 1" class="Bool (strict)"("Colors [4]"=cluster{u32, u32}[] [{9567230, 3381759}]) -> ()  [unwired: 2 in, 2 out]
      }
      frame "111" {
        n405 = property on="Living Room Light 1" class="Bool (strict)"("Colors [4]"=cluster{u32, u32}[] [{16711680, 10420224}]) -> ()  [unwired: 2 in, 2 out]
      }
    }
    n406 = Concatenate Strings(w116, w115) -> (w113:string)
    n407 = case shown="\"110\"" w113 {
      frame "False", Default {
        n408 = property on="Boolean" class="Bool (strict)"() -> ("Colors [4]"=w312:cluster{u32, u32}[])  [unwired: 2 in, 2 out]
        n409 = property on="Master Bedroom Light 2" class="Bool (strict)"("Colors [4]"=w312) -> ()  [unwired: 2 in, 2 out]
      }
      frame "101" {
        n410 = property on="Master Bedroom Light 2" class="Bool (strict)"("Colors [4]"=cluster{u32, u32}[] [{16711680, 10420224}]) -> ()  [unwired: 2 in, 2 out]
      }
      frame "110" {
        n411 = property on="Master Bedroom Light 2" class="Bool (strict)"("Colors [4]"=cluster{u32, u32}[] [{9567230, 3381759}]) -> ()  [unwired: 2 in, 2 out]
      }
      frame "111" {
        n412 = property on="Master Bedroom Light 2" class="Bool (strict)"("Colors [4]"=cluster{u32, u32}[] [{16711680, 10420224}]) -> ()  [unwired: 2 in, 2 out]
      }
    }
    n413 = case shown="\"111\"" w112 {
      frame "False", Default {
        n414 = property on="Boolean" class="Bool (strict)"() -> ("Colors [4]"=w316:cluster{u32, u32}[])  [unwired: 2 in, 2 out]
        n415 = property on="Master Bedroom Light 1" class="Bool (strict)"("Colors [4]"=w316) -> ()  [unwired: 2 in, 2 out]
      }
      frame "101" {
        n416 = property on="Master Bedroom Light 1" class="Bool (strict)"("Colors [4]"=cluster{u32, u32}[] [{16711680, 10420224}]) -> ()  [unwired: 2 in, 2 out]
      }
      frame "110" {
        n417 = property on="Master Bedroom Light 1" class="Bool (strict)"("Colors [4]"=cluster{u32, u32}[] [{9567230, 3381759}]) -> ()  [unwired: 2 in, 2 out]
      }
      frame "111" {
        n418 = property on="Master Bedroom Light 1" class="Bool (strict)"("Colors [4]"=cluster{u32, u32}[] [{16711680, 10420224}]) -> ()  [unwired: 2 in, 2 out]
      }
    }
    n419 = case shown="\"101\"" w25 {
      frame "False", Default {
        n420 = property on="Boolean" class="Bool (strict)"() -> ("Colors [4]"=w288:cluster{u32, u32}[])  [unwired: 2 in, 2 out]
        n421 = property on="Kitchen Light 1" class="Bool (strict)"("Colors [4]"=w288) -> ()  [unwired: 2 in, 2 out]
      }
      frame "101" {
        n422 = property on="Kitchen Light 1" class="Bool (strict)"("Colors [4]"=cluster{u32, u32}[] [{16711680, 10420224}]) -> ()  [unwired: 2 in, 2 out]
      }
      frame "110" {
        n423 = property on="Kitchen Light 1" class="Bool (strict)"("Colors [4]"=cluster{u32, u32}[] [{9567230, 3381759}]) -> ()  [unwired: 2 in, 2 out]
      }
      frame "111" {
        n424 = property on="Kitchen Light 1" class="Bool (strict)"("Colors [4]"=cluster{u32, u32}[] [{16711680, 10420224}]) -> ()  [unwired: 2 in, 2 out]
      }
    }
    n425 = local read "Bedroom 1 Light 1 Dim"() -> (w91:bool)
    n426 = local read "Bedroom 1 Temperature"() -> (w92:dbl)
    n427 = local read "Bedroom 2 Temperature"() -> (w12:dbl)
    n428 = local read "Bedroom 2 Light 1 Dim"() -> (w11:bool)
    n429 = local read "Bedroom 2 Light 1"() -> (w10:bool)
    n430 = local read "Bedroom 1 Light 1"() -> (w90:bool)
    n431 = local read "Balcony Temperature"() -> (w16:dbl)
    n432 = local read "Balcony Temperature"() -> (w19:dbl)
    n433 = local read "Balcony Temperature"() -> (w15:dbl)
    n434 = local read "Balcony Light 1 Dim"() -> (w14:bool)
    n435 = local read "Balcony Light 2 Dim"() -> (w17:bool)
    n436 = local read "Balcony Light 3 Dim"() -> (w20:bool)
    n437 = local read "Balcony Light 1"() -> (w13:bool)
    n438 = local read "Balcony Light 3"() -> (w21:bool)
    n439 = local read "Balcony Light 2"() -> (w18:bool)
    n440 = Greater?(x=w15, y=25.0) -> (0:w65:bool)
    n441 = Greater?(x=w92, y=25.0) -> (0:w100:bool)
    n442 = Greater?(x=w12, y=25.0) -> (0:w78:bool)
    n443 = Greater?(x=w16, y=25.0) -> (0:w52:bool)
    n444 = Greater?(x=w19, y=25.0) -> (0:w39:bool)
    n445 = Boolean To (0,1)(Boolean=w13) -> (0, 1=w71:i16)
    n446 = Boolean To (0,1)(Boolean=w90) -> (0, 1=w106:i16)
    n447 = Boolean To (0,1)(Boolean=w10) -> (0, 1=w84:i16)
    n448 = Boolean To (0,1)(Boolean=w14) -> (0, 1=w74:i16)
    n449 = Boolean To (0,1)(Boolean=w18) -> (0, 1=w58:i16)
    n450 = Boolean To (0,1)(Boolean=w91) -> (0, 1=w109:i16)
    n451 = Boolean To (0,1)(Boolean=w11) -> (0, 1=w87:i16)
    n452 = Boolean To (0,1)(Boolean=w65) -> (0, 1=w70:i16)
    n453 = Boolean To (0,1)(Boolean=w100) -> (0, 1=w105:i16)
    n454 = Boolean To (0,1)(Boolean=w78) -> (0, 1=w83:i16)
    n455 = Boolean To (0,1)(Boolean=w17) -> (0, 1=w61:i16)
    n456 = Boolean To (0,1)(Boolean=w52) -> (0, 1=w57:i16)
    n457 = Boolean To (0,1)(Boolean=w21) -> (0, 1=w45:i16)
    n458 = Boolean To (0,1)(Boolean=w20) -> (0, 1=w48:i16)
    n459 = Boolean To (0,1)(Boolean=w39) -> (0, 1=w44:i16)
    n460 = Number To Decimal String(number=w71, width (-)=i16 1) -> (decimal integer string=w68:string)
    n461 = Number To Decimal String(number=w106, width (-)=i16 1) -> (decimal integer string=w103:string)
    n462 = Number To Decimal String(number=w84, width (-)=i16 1) -> (decimal integer string=w81:string)
    n463 = Number To Decimal String(number=w58, width (-)=i16 1) -> (decimal integer string=w55:string)
    n464 = Number To Decimal String(number=w70, width (-)=i16 1) -> (decimal integer string=w66:string)
    n465 = Number To Decimal String(number=w105, width (-)=i16 1) -> (decimal integer string=w101:string)
    n466 = Number To Decimal String(number=w83, width (-)=i16 1) -> (decimal integer string=w79:string)
    n467 = Number To Decimal String(number=w74, width (-)=i16 1) -> (decimal integer string=w69:string)
    n468 = Number To Decimal String(number=w109, width (-)=i16 1) -> (decimal integer string=w104:string)
    n469 = Number To Decimal String(number=w87, width (-)=i16 1) -> (decimal integer string=w82:string)
    n470 = Number To Decimal String(number=w57, width (-)=i16 1) -> (decimal integer string=w53:string)
    n471 = Number To Decimal String(number=w61, width (-)=i16 1) -> (decimal integer string=w56:string)
    n472 = Number To Decimal String(number=w45, width (-)=i16 1) -> (decimal integer string=w42:string)
    n473 = Number To Decimal String(number=w44, width (-)=i16 1) -> (decimal integer string=w40:string)
    n474 = Number To Decimal String(number=w48, width (-)=i16 1) -> (decimal integer string=w43:string)
    n475 = Concatenate Strings(w68, w69) -> (w67:string)
    n476 = Concatenate Strings(w103, w104) -> (w102:string)
    n477 = Concatenate Strings(w81, w82) -> (w80:string)
    n478 = Concatenate Strings(w55, w56) -> (w54:string)
    n479 = Concatenate Strings(w42, w43) -> (w41:string)
    n480 = Concatenate Strings(w67, w66) -> (w64:string)
    n481 = Concatenate Strings(w102, w101) -> (w99:string)
    n482 = Concatenate Strings(w80, w79) -> (w77:string)
    n483 = Concatenate Strings(w54, w53) -> (w51:string)
    n484 = Concatenate Strings(w41, w40) -> (w38:string)
    n485 = case shown="\"False\", Default" w64 {
      frame "False", Default {
        n486 = property on="Boolean" class="Bool (strict)"() -> ("Colors [4]"=w300:cluster{u32, u32}[])  [unwired: 2 in, 2 out]
        n487 = property on="Balcony Light 1" class="Bool (strict)"("Colors [4]"=w300) -> ()  [unwired: 2 in, 2 out]
      }
      frame "101" {
        n488 = property on="Balcony Light 1" class="Bool (strict)"("Colors [4]"=cluster{u32, u32}[] [{16711680, 10420224}]) -> ()  [unwired: 2 in, 2 out]
      }
      frame "110" {
        n489 = property on="Balcony Light 1" class="Bool (strict)"("Colors [4]"=cluster{u32, u32}[] [{9567230, 3381759}]) -> ()  [unwired: 2 in, 2 out]
      }
      frame "111" {
        n490 = property on="Balcony Light 1" class="Bool (strict)"("Colors [4]"=cluster{u32, u32}[] [{16711680, 10420224}]) -> ()  [unwired: 2 in, 2 out]
      }
    }
    n491 = case shown="\"110\"" w99 {
      frame "False", Default {
        n492 = property on="Boolean" class="Bool (strict)"() -> ("Colors [4]"=w308:cluster{u32, u32}[])  [unwired: 2 in, 2 out]
        n493 = property on="Bedroom 1 Light 1" class="Bool (strict)"("Colors [4]"=w308) -> ()  [unwired: 2 in, 2 out]
      }
      frame "101" {
        n494 = property on="Bedroom 1 Light 1" class="Bool (strict)"("Colors [4]"=cluster{u32, u32}[] [{16711680, 10420224}]) -> ()  [unwired: 2 in, 2 out]
      }
      frame "110" {
        n495 = property on="Bedroom 1 Light 1" class="Bool (strict)"("Colors [4]"=cluster{u32, u32}[] [{9567230, 3381759}]) -> ()  [unwired: 2 in, 2 out]
      }
      frame "111" {
        n496 = property on="Bedroom 1 Light 1" class="Bool (strict)"("Colors [4]"=cluster{u32, u32}[] [{16711680, 10420224}]) -> ()  [unwired: 2 in, 2 out]
      }
    }
    n497 = case shown="\"False\", Default" w77 {
      frame "False", Default {
        n498 = property on="Boolean" class="Bool (strict)"() -> ("Colors [4]"=w304:cluster{u32, u32}[])  [unwired: 2 in, 2 out]
        n499 = property on="Bedroom 2 Light 1" class="Bool (strict)"("Colors [4]"=w304) -> ()  [unwired: 2 in, 2 out]
      }
      frame "101" {
        n500 = property on="Bedroom 2 Light 1" class="Bool (strict)"("Colors [4]"=cluster{u32, u32}[] [{16711680, 10420224}]) -> ()  [unwired: 2 in, 2 out]
      }
      frame "110" {
        n501 = property on="Bedroom 2 Light 1" class="Bool (strict)"("Colors [4]"=cluster{u32, u32}[] [{9567230, 3381759}]) -> ()  [unwired: 2 in, 2 out]
      }
      frame "111" {
        n502 = property on="Bedroom 2 Light 1" class="Bool (strict)"("Colors [4]"=cluster{u32, u32}[] [{16711680, 10420224}]) -> ()  [unwired: 2 in, 2 out]
      }
    }
    n503 = case shown="\"False\", Default" w51 {
      frame "False", Default {
        n504 = property on="Boolean" class="Bool (strict)"() -> ("Colors [4]"=w296:cluster{u32, u32}[])  [unwired: 2 in, 2 out]
        n505 = property on="Balcony Light 2" class="Bool (strict)"("Colors [4]"=w296) -> ()  [unwired: 2 in, 2 out]
      }
      frame "101" {
        n506 = property on="Balcony Light 2" class="Bool (strict)"("Colors [4]"=cluster{u32, u32}[] [{16711680, 10420224}]) -> ()  [unwired: 2 in, 2 out]
      }
      frame "110" {
        n507 = property on="Balcony Light 2" class="Bool (strict)"("Colors [4]"=cluster{u32, u32}[] [{9567230, 3381759}]) -> ()  [unwired: 2 in, 2 out]
      }
      frame "111" {
        n508 = property on="Balcony Light 2" class="Bool (strict)"("Colors [4]"=cluster{u32, u32}[] [{16711680, 10420224}]) -> ()  [unwired: 2 in, 2 out]
      }
    }
    n509 = case shown="\"False\", Default" w38 {
      frame "False", Default {
        n510 = property on="Boolean" class="Bool (strict)"() -> ("Colors [4]"=w292:cluster{u32, u32}[])  [unwired: 2 in, 2 out]
        n511 = property on="Balcony Light 3" class="Bool (strict)"("Colors [4]"=w292) -> ()  [unwired: 2 in, 2 out]
      }
      frame "101" {
        n512 = property on="Balcony Light 3" class="Bool (strict)"("Colors [4]"=cluster{u32, u32}[] [{16711680, 10420224}]) -> ()  [unwired: 2 in, 2 out]
      }
      frame "110" {
        n513 = property on="Balcony Light 3" class="Bool (strict)"("Colors [4]"=cluster{u32, u32}[] [{9567230, 3381759}]) -> ()  [unwired: 2 in, 2 out]
      }
      frame "111" {
        n514 = property on="Balcony Light 3" class="Bool (strict)"("Colors [4]"=cluster{u32, u32}[] [{16711680, 10420224}]) -> ()  [unwired: 2 in, 2 out]
      }
    }
  }
  n515 = TCP Close Connection "TCP Close \nConnection"(connection ID=w5, error in (no error)=w3) -> (error out=w2:errorcluster)  [unwired: 1 in, 1 out]
  n516 = call <vilib>:"Clear Errors.vi"("error in (no error)"=w2) -> ()  [unwired: 5 in, 2 out]
  "Boolean" <- TRUE ("Boolean")
